vi "Sub Initialize.vi"(8 "error in (no error)":errorcluster, 11 "Instrument Recorder in":refnum<class "Pulse Recorder.lvclass">) -> (0 "error out":errorcluster, 2 "Initialize Result":refnum<class "Acquired Result.lvclass">, 3 "Instrument Recorder out":refnum<class "Pulse Recorder.lvclass">)   [LabVIEW 2016, in "Pulse Recorder.lvclass"]
uses:
  Pulse Recorder.lvclass
  NHMFL_Core/Libraries/Instruments/Results/Acquired Result/Acquired Result.lvclass
  Pulse Recorder.lvclass/Pulse Recorder.ctl
  Instrument Actor/Instrument Actor.lvclass
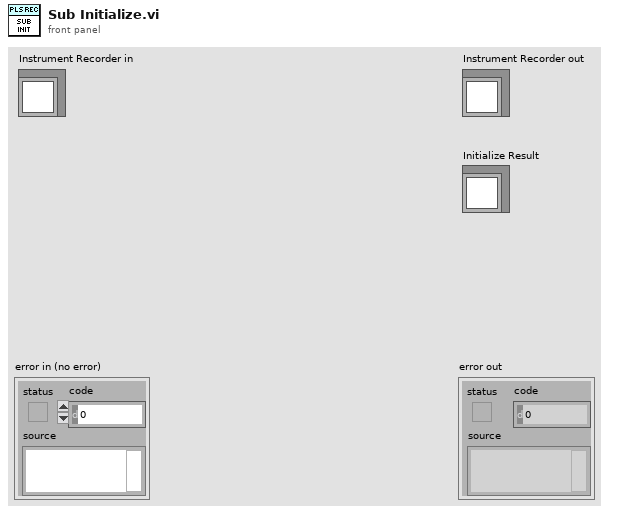
[diagram p1: front panel]
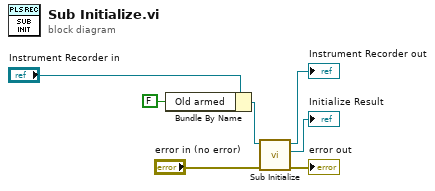
[diagram p0: block diagram]
diagram:
  n1 = Bundle By Name(cluster="Instrument Recorder in", "Old armed"=FALSE ("Armed")) -> (w1:refnum<class "Pulse Recorder.lvclass">)
  n2 = call-parent "Sub Initialize.vi"("error in (no error)"="error in (no error)", "Instrument Recorder in"=w1) -> ("error out"=→"error out":errorcluster, "Initialize Result"=→"Initialize Result":refnum<class "Acquired Result.lvclass">, "Instrument Recorder out"=→"Instrument Recorder out":refnum<class "Pulse Recorder.lvclass">)  [unwired: 7 in]
